vi "gm_measuringpoint_valves_feedback.vi"(10 "Output - Cluster gas":T1 {"GM TS-2[°C]" format="%.2g"; "GM TS-1 [°C]" format="%.2g"; "GM DS-1 [bar]" format="%.4g"; "GM DS-2 [bar]" format="%.4g"; "GM GZ-1 [imp]" format="%.2g"; "GA1 h2 [%]" format="%.2g"; "GA1 co2 [%]" format="%.2g"; "GA1 ch4 [%]" format="%.2g"}, 11 "measuring point":u32) -> (3 "measuring point":u32)   [LabVIEW 2011]
uses:
  Output - Cluster gas.ctl
  gas_values.ctl
panel:
  out "number":u32
  # "qualitätsmessung"
  # "quantitätsmessung"
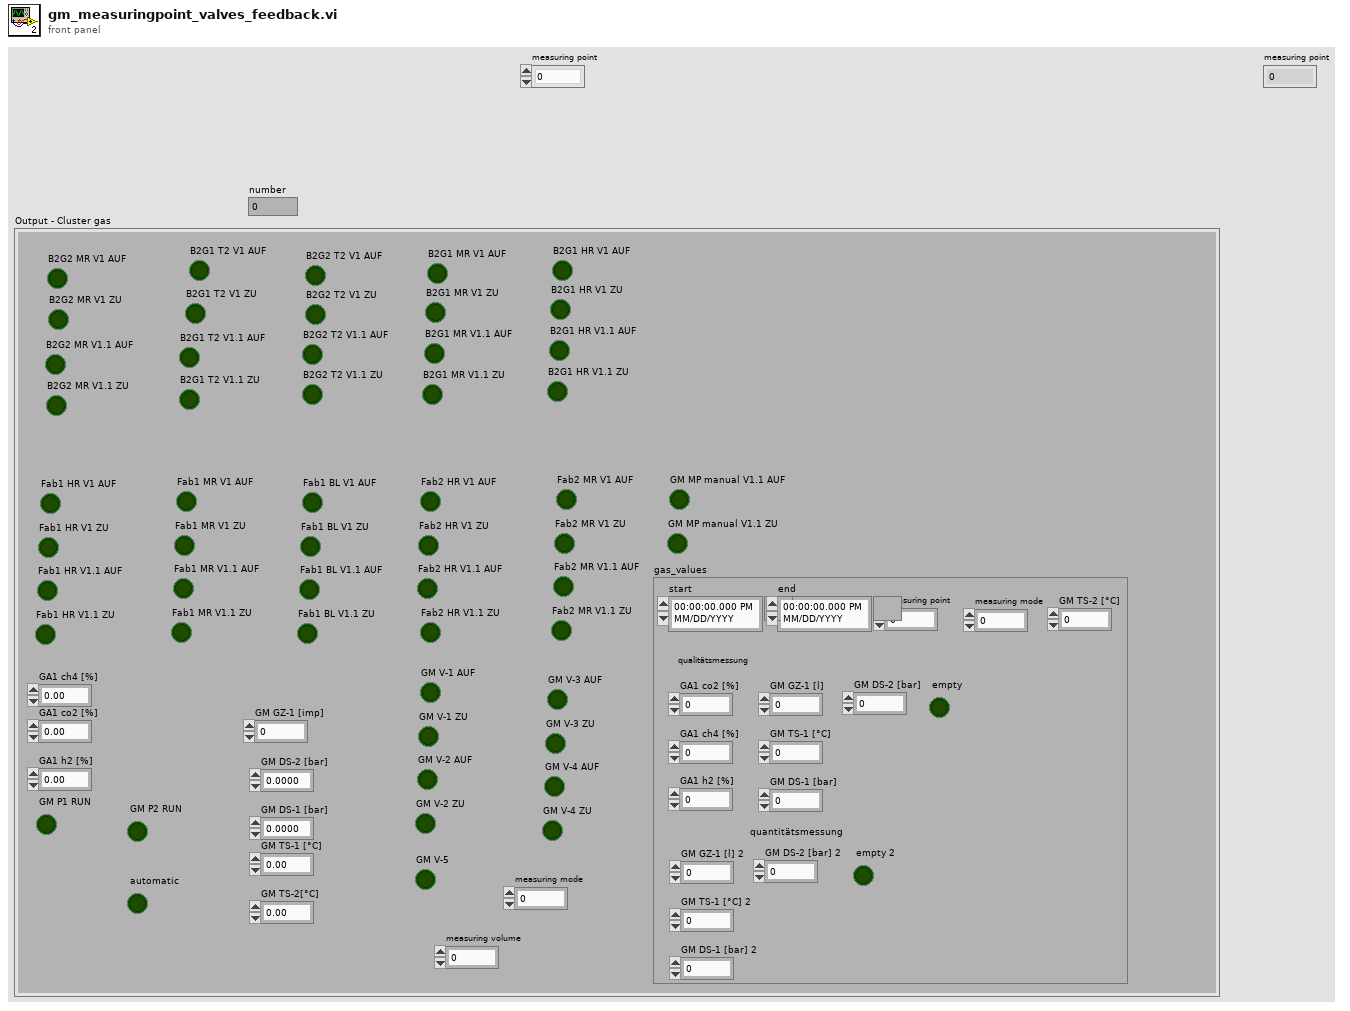
[diagram p1: front panel]
types:
  T1 = typedef "Output - Cluster gas.ctl" = cluster{"B2G2 MR V1.1 AUF":bool, "B2G2 MR V1.1 ZU":bool, "B2G2 MR V1 AUF":bool, "B2G2 MR V1 ZU":bool, "B2G1 T2 V1 AUF":bool, "B2G1 T2 V1 ZU":bool, "B2G1 T2 V1.1 AUF":bool, "B2G1 T2 V1.1 ZU":bool, "B2G2 T2 V1 AUF":bool, "B2G2 T2 V1 ZU":bool, "B2G2 T2 V1.1 ZU":bool, "B2G2 T2 V1.1 AUF":bool, "B2G1 MR V1 AUF":bool, "B2G1 MR V1 ZU":bool, "B2G1 MR V1.1 AUF":bool, "B2G1 MR V1.1 ZU":bool, "B2G1 HR V1 AUF":bool, "B2G1 HR V1 ZU":bool, "B2G1 HR V1.1 AUF":bool, "B2G1 HR V1.1 ZU":bool, "Fab1 HR V1 AUF":bool, "Fab1 HR V1 ZU":bool, "Fab1 HR V1.1 AUF":bool, "Fab1 HR V1.1 ZU":bool, "Fab1 MR V1 AUF":bool, "Fab1 MR V1 ZU":bool, "Fab1 MR V1.1 AUF":bool, "Fab1 MR V1.1 ZU":bool, "Fab1 BL V1 AUF":bool, "Fab1 BL V1 ZU":bool, "Fab1 BL V1.1 AUF":bool, "Fab1 BL V1.1 ZU":bool, "Fab2 HR V1 AUF":bool, "Fab2 HR V1 ZU":bool, "Fab2 HR V1.1 AUF":bool, "Fab2 HR V1.1 ZU":bool, "Fab2 MR V1 AUF":bool, "Fab2 MR V1 ZU":bool, "Fab2 MR V1.1 AUF":bool, "Fab2 MR V1.1 ZU":bool, "GA1 ch4 [%]":dbl, "GA1 co2 [%]":dbl, "GA1 h2 [%]":dbl, "GM P1 RUN":bool, "GM V-1 AUF":bool, "GM V-1 ZU":bool, "GM V-2 AUF":bool, "GM V-2 ZU":bool, "GM V-3 AUF":bool, "GM V-3 ZU":bool, "GM V-4 AUF":bool, "GM V-4 ZU":bool, "GM P2 RUN":bool, "GM GZ-1 [imp]":u32, "GM DS-2 [bar]":dbl, "GM DS-1 [bar]":dbl, "GM TS-1 [°C]":dbl, "GM TS-2[°C]":dbl, "gas_values":T2, "measuring mode":u8, "GM V-5":bool, "measuring volume":dbl, "automatic":bool, "GM MP manual V1.1 AUF":bool, "GM MP manual V1.1 ZU":bool}
  T2 = typedef "gas_values.ctl" = cluster{"start":timestamp, "GM DS-2 [bar]":dbl, "GA1 ch4 [%]":dbl, "GA1 co2 [%]":dbl, "GA1 h2 [%]":dbl, "GM DS-1 [bar]":dbl, "GM TS-1 [°C]":dbl, "GM TS-2 [°C]":dbl, "GM GZ-1 [l]":dbl, "measuring point":u8, "end":timestamp, "empty":bool, "GM GZ-1 [l] 2":dbl, "GM TS-1 [°C] 2":dbl, "GM DS-1 [bar] 2":dbl, "GM DS-2 [bar] 2":dbl, "empty 2":bool, "measuring mode":u8}
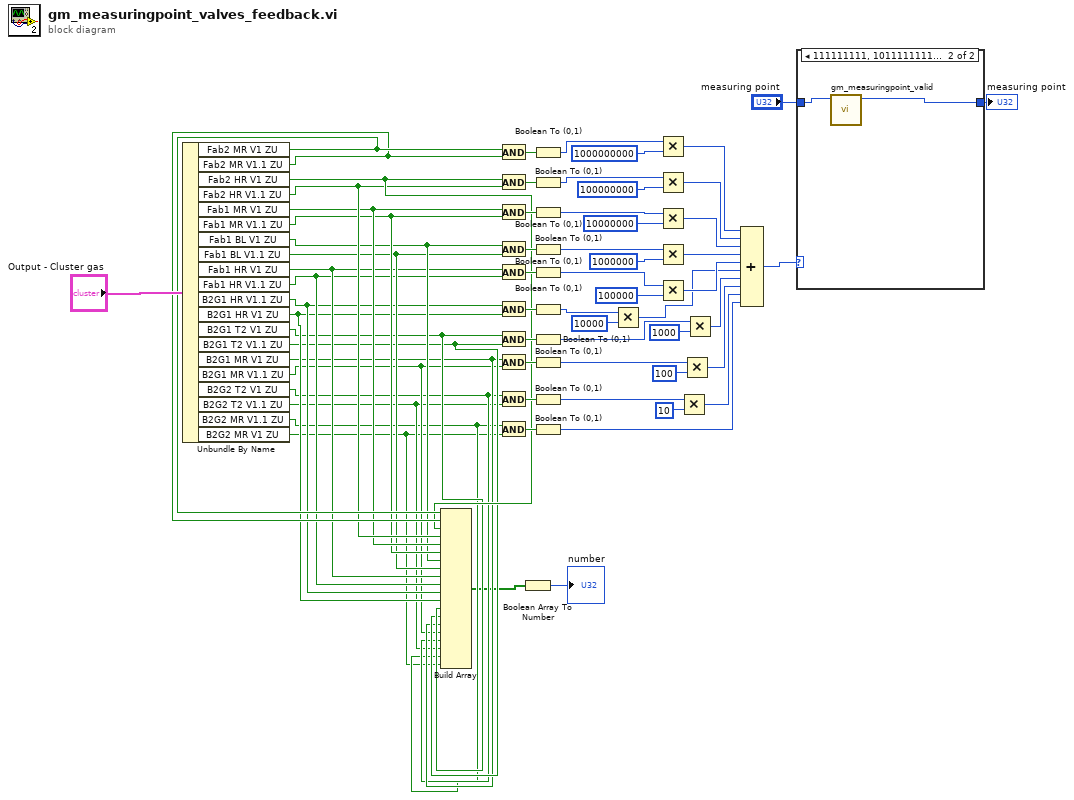
[diagram p0: block diagram]
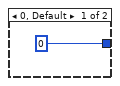
[diagram p2: hidden frame]
diagram:
  n1 = Unbundle By Name("Output - Cluster gas") -> ("Fab2 MR V1 ZU"=w22:bool, "Fab2 MR V1.1 ZU"=w21:bool, "Fab2 HR V1 ZU"=w20:bool, "Fab2 HR V1.1 ZU"=w19:bool, "Fab1 MR V1 ZU"=w18:bool, "Fab1 MR V1.1 ZU"=w17:bool, "Fab1 BL V1 ZU"=w16:bool, "Fab1 BL V1.1 ZU"=w15:bool, "Fab1 HR V1 ZU"=w14:bool, "Fab1 HR V1.1 ZU"=w13:bool, "B2G1 HR V1.1 ZU"=w12:bool, "B2G1 HR V1 ZU"=w11:bool, "B2G1 T2 V1 ZU"=w10:bool, "B2G1 T2 V1.1 ZU"=w9:bool, "B2G1 MR V1 ZU"=w8:bool, "B2G1 MR V1.1 ZU"=w7:bool, "B2G2 T2 V1 ZU"=w6:bool, "B2G2 T2 V1.1 ZU"=w5:bool, "B2G2 MR V1.1 ZU"=w4:bool, "B2G2 MR V1 ZU"=w3:bool)
  n2 = Build Array(w22, w21, w20, w19, w18, w17, w16, w15, w14, w13, w12, w11, w10, w9, w8, w7, w6, w5, w4, w3) -> (w2:bool[])
  n3 = And(x=w22, y=w21) -> (x .and. y?=w27:bool)
  n4 = And(x=w20, y=w19) -> (x .and. y?=w28:bool)
  n5 = And(x=w18, y=w17) -> (x .and. y?=w36:bool)
  n6 = And(x=w16, y=w15) -> (x .and. y?=w35:bool)
  n7 = And(x=w14, y=w13) -> (x .and. y?=w34:bool)
  n8 = And(x=w12, y=w11) -> (x .and. y?=w33:bool)
  n9 = And(x=w10, y=w9) -> (x .and. y?=w32:bool)
  n10 = And(x=w8, y=w7) -> (x .and. y?=w31:bool)
  n11 = And(x=w6, y=w5) -> (x .and. y?=w30:bool)
  n12 = And(x=w4, y=w3) -> (x .and. y?=w29:bool)
  n13 = Boolean Array To Number(Boolean array=w2) -> (number=→"number":u32)
  n14 = Boolean To (0,1)(Boolean=w27) -> (0, 1=w57:i16)
  n15 = Boolean To (0,1)(Boolean=w28) -> (0, 1=w56:i16)
  n16 = Boolean To (0,1)(Boolean=w36) -> (0, 1=w55:i16)
  n17 = Boolean To (0,1)(Boolean=w35) -> (0, 1=w54:i16)
  n18 = Boolean To (0,1)(Boolean=w34) -> (0, 1=w53:i16)
  n19 = Boolean To (0,1)(Boolean=w33) -> (0, 1=w52:i16)
  n20 = Boolean To (0,1)(Boolean=w32) -> (0, 1=w44:i16)
  n21 = Boolean To (0,1)(Boolean=w31) -> (0, 1=w41:i16)
  n22 = Boolean To (0,1)(Boolean=w30) -> (0, 1=w38:i16)
  n23 = Boolean To (0,1)(Boolean=w29) -> (0, 1=w37:i16)
  n24 = Multiply(x=w52, y=u64 10000) -> (x*y=w24:u64)
  n25 = Multiply(x=w57, y=u64 1000000000) -> (x*y=w62:u64)
  n26 = Multiply(x=w56, y=u64 100000000) -> (x*y=w61:u64)
  n27 = Multiply(x=w55, y=u64 10000000) -> (x*y=w60:u64)
  n28 = Multiply(x=w54, y=u64 1000000) -> (x*y=w59:u64)
  n29 = Multiply(x=w53, y=u64 100000) -> (x*y=w58:u64)
  n30 = Multiply(x=w38, y=u64 10) -> (x*y=w39:u64)
  n31 = Multiply(x=w41, y=u64 100) -> (x*y=w43:u64)
  n32 = Multiply(x=w44, y=u64 1000) -> (x*y=w25:u64)
  n33 = Compound Arithmetic op=ADD(w62, w61, w60, w59, w58, w24, w25, w43, w39, w37) -> (w63:u64)
  n34 = case shown="111111111, 1011111111, 1101111111, 1110111111, 1111011111, 1111101111, 1111110111, 1111111011, 1111111101, 1111111110, 1111111111" w63 {
    tunnel: "measuring point" -> [_ w67]
    tunnel: [u32 0 ("measuring point") w66] -> w23
    frame 0, Default {
    }
    frame 111111111, 1011111111, 1101111111, 1110111111, 1111011111, 1111101111, 1111110111, 1111111011, 1111111101, 1111111110, 1111111111 {
      n35 = call "gm_measuringpoint_valid.vi"("measuring point in"=w67) -> ("measuring point out"=w66:u32)  [unwired: 9 in, 1 out]
    }
  }
  "measuring point" <- w23
